vi "MHTL VBS CREATOR.vi"(8 "error in (no error)":errorcluster, 9 "mht dest path":path, 10 "htm path":path, 11 "script path":path=path "C:/Development/SI.LIB/HTML/MHTML/mht_converter.vbs") -> (0 "error out":errorcluster)   [LabVIEW 2011]
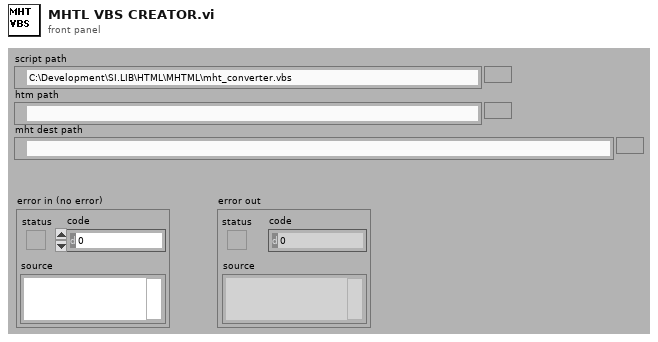
[diagram p1: front panel]
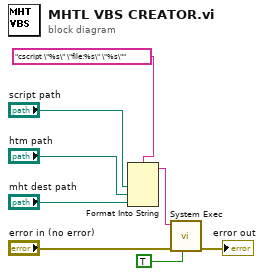
[diagram p0: block diagram]
diagram:
  n1 = Format Into String(format string="cscript \"%s\" \"file:%s\" \"%s\"", "script path", "htm path", "mht dest path") -> (resulting string=w8:string)  [unwired: 2 in, 1 out]
  n2 = call <vilib>:"System Exec.vi"("run minimized? (F)"=TRUE, "error in (no error)"="error in (no error)", "command line"=w8) -> ("error out"=→"error out":errorcluster)  [unwired: 5 in, 3 out]
